vi "is Running.vi"(11 "TriggerAction in":refnum<class "TriggerAction Q.lvclass">) -> (2 "Running?":bool, 3 "TriggerAction out":refnum<class "TriggerAction Q.lvclass">)   [LabVIEW 2016, in "TriggerAction Q.lvclass"]
uses:
  <userlib>/Common Components/TriggerAction Q/TriggerAction Q/TriggerAction Q.lvclass
  <userlib>/Common Components/TriggerAction Q/TriggerAction Q/TriggerAction Q.lvclass/TriggerAction Q.ctl
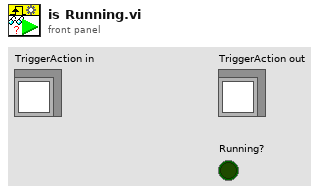
[diagram p1: front panel]
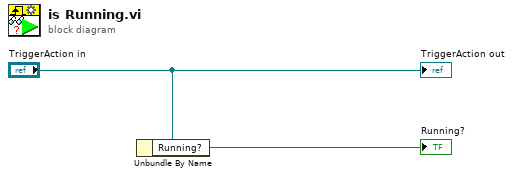
[diagram p0: block diagram]
diagram:
  n1 = Unbundle By Name("TriggerAction in") -> ("Running?"=→"Running?":bool)
  "TriggerAction out" <- "TriggerAction in"
